vi "Write states.vi"(8 "error in (no error)":errorcluster, 10 "states":T1, 11 "NewTestTactic in":refnum<class "NewTestTactic.lvclass">) -> (0 "error out":errorcluster, 3 "NewTestTactic out":refnum<class "NewTestTactic.lvclass">)   [LabVIEW 2022 SP3, in "NewTestTactic.lvclass"]
uses:
  NewTestTactic.lvclass
  Control 1.ctl
  NewTestTactic.lvclass/NewTestTactic.ctl
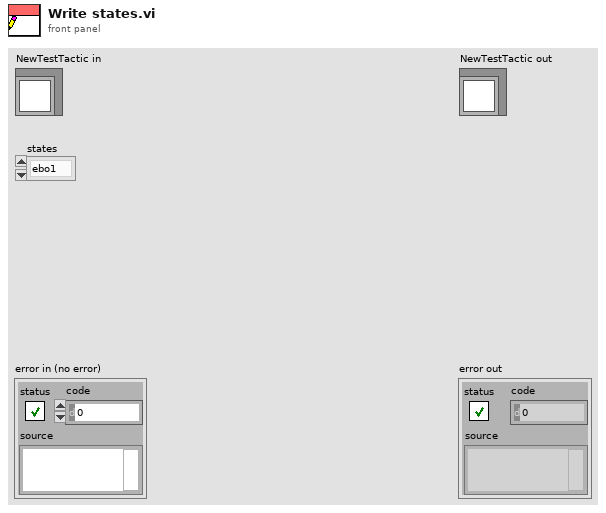
[diagram p1: front panel]
types:
  T1 = typedef "Control 1.ctl" = enum16{"ebo1", "ebo2", "bo3"}
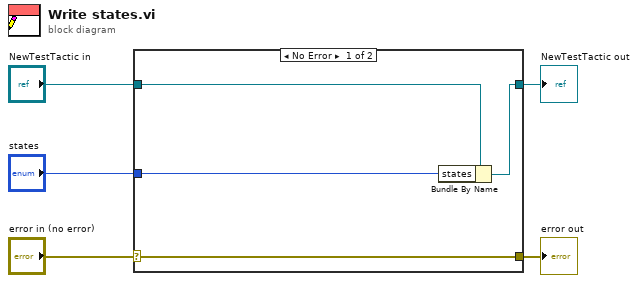
[diagram p0: block diagram]
diagram:
  n1 = case shown="No Error" "error in (no error)" {
    selector: "error in (no error)" -> [w9 w10]
    tunnel: [w9 w10] -> w4
    tunnel: [w7 w11] -> w2
    tunnel: "NewTestTactic in" -> [w8 w11]
    tunnel: "states" -> [w6 _]
    frame No Error {
      n2 = Bundle By Name(cluster=w8, "states"=w6) -> (w7:refnum<class "NewTestTactic.lvclass">)
    }
    frame Error {
    }
  }
  "error out" <- w4
  "NewTestTactic out" <- w2
